vi "AssertEqual_Tests.vi"(11 "error in (no error)":errorcluster) -> (15 "error out":errorcluster)   [LabVIEW 2016, in "DronaTest.lvlib"]
uses:
  DronaTest.lvlib
  APIs/Assert/AssertControlValue/Equal.vi
  <vilib>/addons/_JKI Toolkits/Caraya/classes/Assert/Assert Error.vi
  <vilib>/addons/_JKI Toolkits/Caraya/classes/Assert/Assert Equal Value_Variant.vi
  <vilib>/addons/_JKI Toolkits/Caraya/classes/Test/Test.lvclass
  Drona.lvlib
  <vilib>/addons/_JKI Toolkits/Caraya/classes/Assert/Assert.lvclass
  APIs/Assert/AssertControlValue/AssertControlValue.lvlib
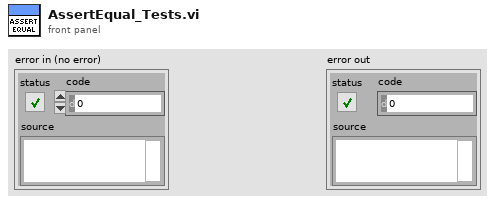
[diagram p1: front panel]
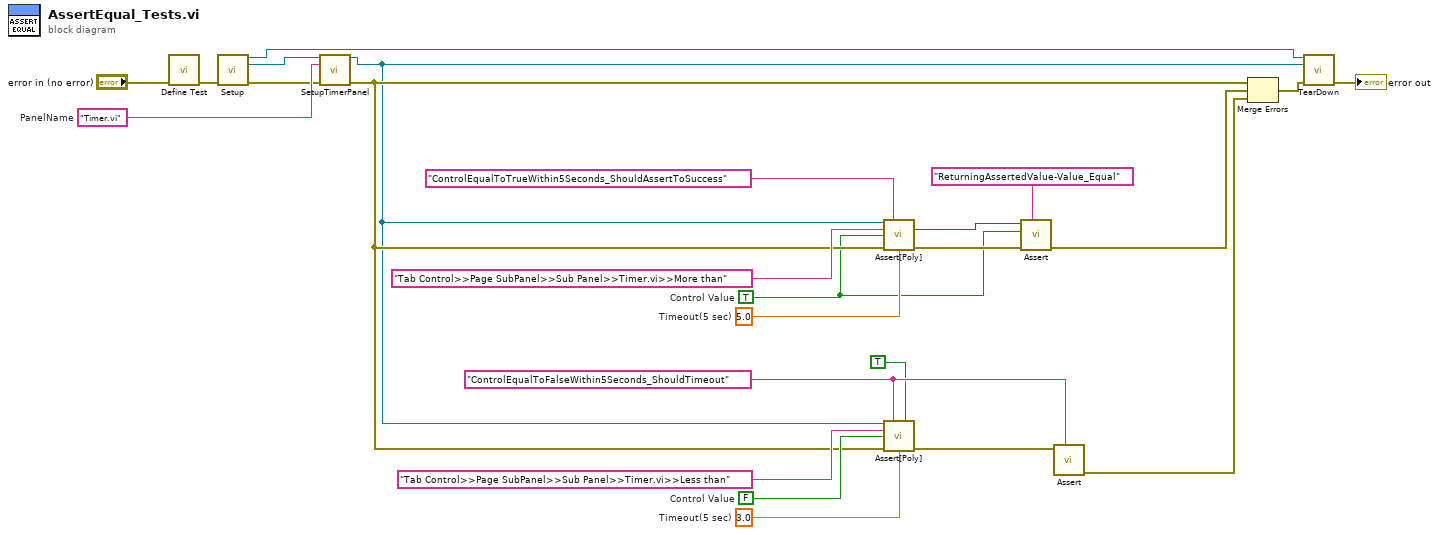
[diagram p0: block diagram]
diagram:
  w15 = "Timer.vi"  # PanelName
  w24 = FALSE  # Control Value
  w21 = 3.0  # Timeout(5 sec)
  w20 = "ControlEqualToFalseWithin5Seconds_ShouldTimeout" ("string")
  w22 = 5.0  # Timeout(5 sec)
  w2 = TRUE  # Control Value
  n1 = call <vilib>:"Define Test.vi"("error in (no error)"="error in (no error)") -> ("error out"=w12:errorcluster)  [unwired: 9 in, 1 out]
  n2 = call "Setup.vi"("error in (no error)"=w12) -> ("Application Ref"=w9:refnum<vi>, "VI out"=w13:refnum<vi>, "error out"=w14:errorcluster)  [unwired: 12 in]
  n3 = call "SetupTimerPanel.vi"("VI in"=w13, "Panel Name"=w15, "error in (no error)"=w14) -> ("VI out"=w7:refnum<vi>, "error out"=w8:errorcluster)  [unwired: 11 in]
  n4 = call-poly "Assert[Poly].vi"("VI Reference In"=w7, "Test Label"="ControlEqualToTrueWithin5Seconds_ShouldAssertToSuccess" ("string"), "Control Path"="Tab Control>>Page SubPanel>>Sub Panel>>Timer.vi>>More than", "Control Value"=w2, "Error In"=w8, "Timeout(5 sec)"=w22) -> ("Asserted Value"=w3:variant, "Error Out"=w5:errorcluster)  [unwired: 7 in, 1 out]
  n5 = call-poly "Assert[Poly].vi"("VI Reference In"=w7, "Test Label"=w20, "Assert Only? (F)"=TRUE, "Control Path"="Tab Control>>Page SubPanel>>Sub Panel>>Timer.vi>>Less than", "Control Value"=w24, "Error In"=w8, "Timeout(5 sec)"=w21) -> ("Error Out"=w19:errorcluster)  [unwired: 6 in, 2 out]
  n6 = call-poly <vilib>:"Assert.vi"("Label"="ReturningAssertedValue-Value_Equal", "error in (no error)"=w5, "Y"=w2, "X"=w3) -> ("error out"=w4:errorcluster)  [unwired: 6 in, 1 out]
  n7 = call-poly <vilib>:"Assert.vi"("Label"=w20, "Error?"=w19) -> ("error out"=w16:errorcluster)  [unwired: 8 in, 1 out]
  n8 = Merge Errors(w8, w4, w16) -> (w11:errorcluster)
  n9 = call "TearDown.vi"("Application Ref"=w9, "VI in"=w7, "error in (no error)"=w11) -> ("error out"=→"error out":errorcluster)  [unwired: 12 in]
